vi "Between.vi"(9 "Hallway Position in":i32, 10 "Room in":string, 11 "Position in":i32) -> (0 "Betwwen?":bool, 1 "Hallway Position out":i32, 2 "Room out":string, 3 "Position out":i32)   [LabVIEW 2019, in "23.lvlib" / "State.lvclass"]
uses:
  State.lvclass
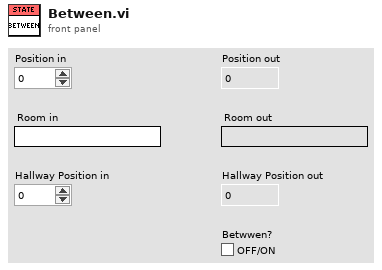
[diagram p1: front panel]
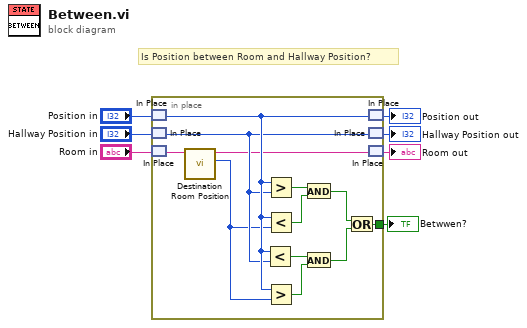
[diagram p0: block diagram]
diagram:
  # "Is Position between Room and Hallway Position?"
  n1 = in-place {
    in-place-border: [w19] -> w7
    n2 = in-place-match #1("Position in") -> (w12:i32)
    n3 = in-place-match #2("Hallway Position in") -> (w10:i32)
    n4 = in-place-match #3("Room in") -> (w11:string)
    n5 = call "Destination Room Position.vi"("Amphipod Type in"=w11) -> ("Destination Room Position"=w9:i32, "Amphipod Type out"=w8:string)  [unwired: 9 in]
    n6 = Less?(x=w12, y=w10) -> (x < y?=w13:bool)
    n7 = Greater?(x=w12, y=w10) -> (0:w15:bool)
    n8 = Less?(x=w12, y=w9) -> (x < y?=w16:bool)
    n9 = Greater?(x=w12, y=w9) -> (0:w14:bool)
    n10 = And(x=w15, y=w16) -> (x .and. y?=w17:bool)
    n11 = And(x=w13, y=w14) -> (x .and. y?=w18:bool)
    n12 = Or(x=w17, y=w18) -> (x .or. y?=w19:bool)
    n13 = in-place-match #1(w12) -> (→"Position out":i32)
    n14 = in-place-match #2(w10) -> (→"Hallway Position out":i32)
    n15 = in-place-match #3(w8) -> (→"Room out":string)
  }
  "Betwwen?" <- w7
